vi "scanning_template_5_24.vi"() -> ()   [LabVIEW 2022 SP3]
uses:
  <vilib>/Utility/file.llb/Write Delimited Spreadsheet (string).vi
panel:
  in  "Backwards x":bool
  in  "ms to wait after move":u32=200
  in  "ANC300 address":refnum<visa-resource-name>="COM8"
  in  "Snake":bool
  in  "File to save to":path=path "C:/Users/Public/OneDrive/Desktop/test.txt"
  in  "Select Scan Type":u16(ring) items=["line scan", "rectangular scan"]
  in  "scan points":i32
  in  "y end":i32
  in  "x end":i32
  in  "y start":i32
  in  "x start":i32
  in  "y scan points":i32
  in  "x scan points":i32
  in  "y scan size":i32
  in  "x scan size":i32
  in  "y center":i32
  in  "x center":i32
  # "Scaning Setup"
  # "Rectangular Scan Parameters"
  # "Line Scan Parameters"
  # "Measurement Setup"
  # "insert measurement controls"
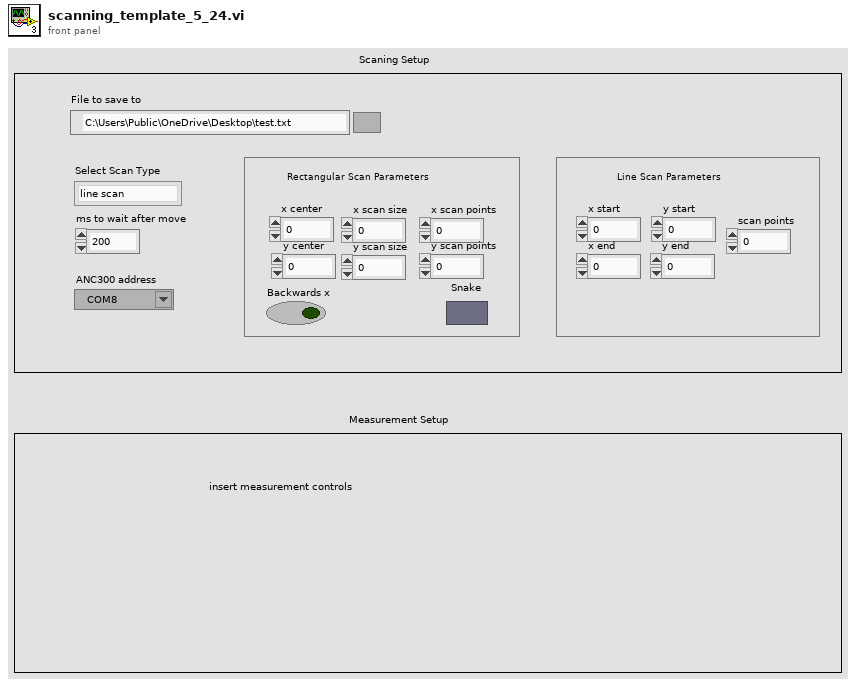
[diagram p1: front panel]
types:
  T1 = cluster{"error ":bool, "error number":i32, "error code":string}
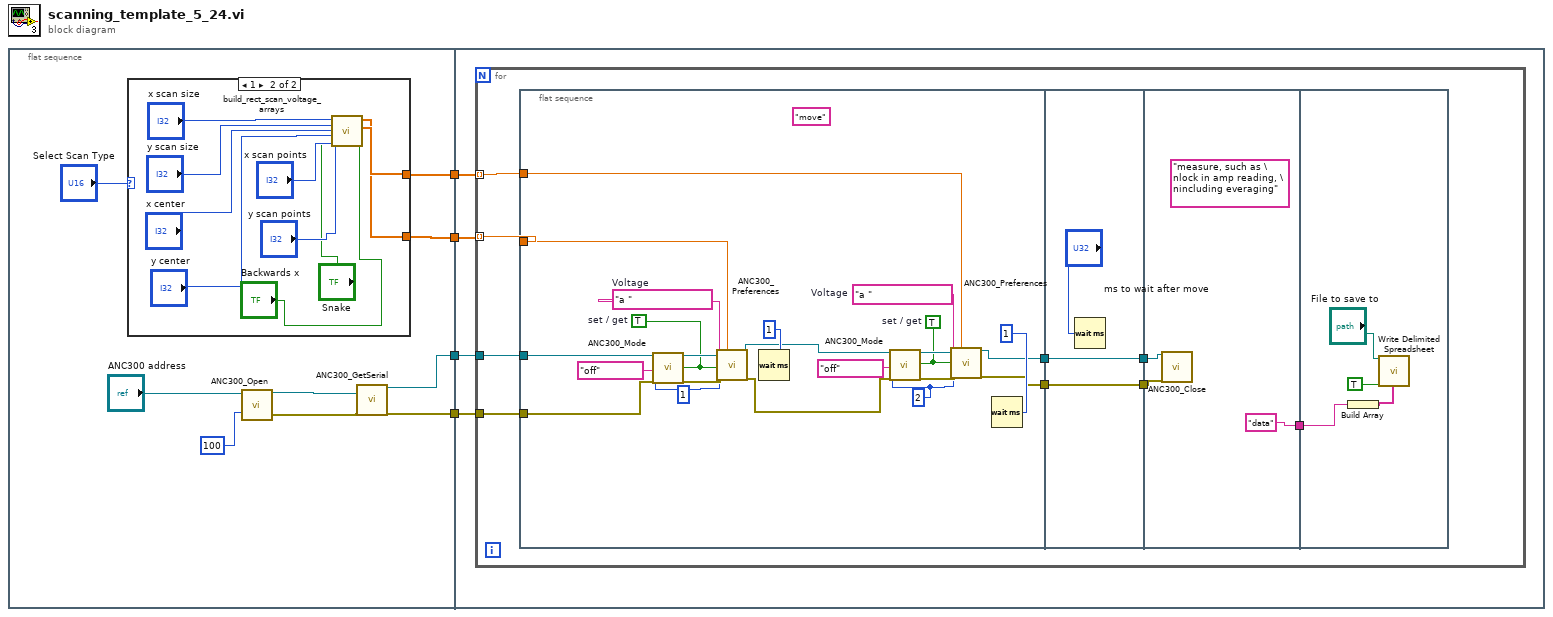
[diagram p0: block diagram]
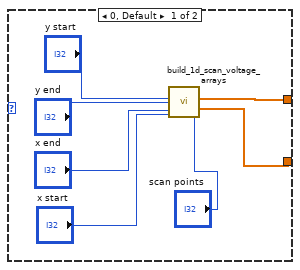
[diagram p2: hidden frame]
diagram:
  n1 = flat-sequence {
    tunnel: [w12] -> w4
    tunnel: [w13] -> w3
    tunnel: [w7] -> w2
    tunnel: [w6] -> w1
    tunnel: w4 -> [w34]
    tunnel: w3 -> [w33]
    tunnel: w2 -> [w32]
    tunnel: w1 -> [w31]
    frame #0 {
      n2 = case shown="1" "Select Scan Type" {
        tunnel: [w14 w30] -> w13
        tunnel: [w15 w29] -> w12
        frame 0, Default {
          n3 = call "build_1d_scan_voltage_arrays.vi"("y end"="y end", "y start"="y start", "scan points"="scan points", "x start"="x start", "x end"="x end") -> ("y voltage array"=w14:dbl[], "x voltage array"=w15:dbl[])  [unwired: 5 in]
        }
        frame 1 {
          n4 = call "build_rect_scan_voltage_arrays.vi"("Backwards x"="Backwards x", "y scan points"="y scan points", "y scan size"="y scan size", "x center"="x center", "Snake"="Snake", "y center"="y center", "x scan points"="x scan points", "x scan size"="x scan size") -> ("y voltage array"=w30:dbl[], "x voltage array"=w29:dbl[])  [unwired: 2 in]
        }
      }
      n5 = call "ANC300_Open.vi"("ANC300 Communication Port In"="ANC300 address", "milliseconds to wait"=u32 100 ("millisecond timer value")) -> ("ANC300 Communication Port Out"=w8:refnum<visa-resource-name>, "error out"=w5:T1)  [unwired: 13 in, 3 out]
      n6 = call "ANC300_GetSerial.vi"("ANC300 Communication Port In"=w8, "error in"=w5) -> ("ANC300 Communication Port Out"=w7:refnum<visa-resource-name>, "error out"=w6:T1)  [unwired: 10 in, 6 out]
    }
    frame #1 {
      n7 = for {
        tunnel: w34 -> [w43] mode=indexing
        tunnel: w33 -> [w42] mode=indexing
        tunnel: w32 -> [w41]
        tunnel: w31 -> [w40]
        n8 = flat-sequence {
          tunnel: w43 -> [w50]
          tunnel: w42 -> [w49]
          tunnel: w41 -> [w52]
          tunnel: w40 -> [w47]
          tunnel: [w45] -> w38
          tunnel: [w44] -> w37
          tunnel: w38 -> [w67]
          tunnel: w37 -> [w66]
          tunnel: [w67] -> w36
          tunnel: [w66] -> w35
          tunnel: ["data"] -> w39
          tunnel: w36 -> [w70]
          tunnel: w35 -> [w69]
          tunnel: w39 -> [w72]
          frame #0 {
            w53 = 2
            w54 = 1
            w55 = TRUE  # set / get
            w57 = "a "  # Voltage
            w60 = TRUE  # set / get
            w63 = "a "  # Voltage
            (unwired) "move"
            n9 = call "ANC300_Mode.vi"("ANC300 Communication Port In"=w52, "Axis"=w54, "axis mode in"="off", "error in"=w47, "set / get"=w60) -> ("ANC300 Communication Port Out"=w65:refnum<visa-resource-name>, "error out"=w64:T1)  [unwired: 8 in, 5 out]
            n10 = call "ANC300_Preferences.vi"("ANC300 Communication Port In"=w65, "Axis"=w54, "value in"=w50, "parameter"=w63, "error in"=w64, "set / get"=w60) -> ("ANC300 Communication Port Out"=w48:refnum<visa-resource-name>, "error out"=w46:T1)  [unwired: 6 in, 6 out]
            n11 = Wait (ms)(milliseconds to wait=u32 1 ("1: ms to wait")) -> ()  [unwired: 1 out]
            n12 = call "ANC300_Mode.vi"("ANC300 Communication Port In"=w48, "Axis"=w53, "axis mode in"="off", "error in"=w46, "set / get"=w55) -> ("ANC300 Communication Port Out"=w59:refnum<visa-resource-name>, "error out"=w58:T1)  [unwired: 8 in, 5 out]
            n13 = call "ANC300_Preferences.vi"("ANC300 Communication Port In"=w59, "Axis"=w53, "value in"=w49, "parameter"=w57, "error in"=w58, "set / get"=w55) -> ("ANC300 Communication Port Out"=w45:refnum<visa-resource-name>, "error out"=w44:T1)  [unwired: 6 in, 6 out]
            n14 = Wait (ms)(milliseconds to wait=u32 1 ("2: ms to wait")) -> ()  [unwired: 1 out]
          }
          frame #1 {
            n15 = Wait (ms)(milliseconds to wait="ms to wait after move") -> ()  [unwired: 1 out]
          }
          frame #2 {
            (unwired) "measure, such as \nlock in amp reading, \nincluding everaging"
            n16 = call "ANC300_Close.vi"("ANC300 Communication Port In"=w70, "error in"=w69) -> ()  [unwired: 17 in, 1 out]
          }
          frame #3 {
            n17 = Build Array(w72) -> (w75:string[])
            n18 = call-poly <vilib>:"Write Delimited Spreadsheet.vi"("file path (dialog if empty)"="File to save to", "1D data"=w75, "append to file? (new file:F)"=TRUE) -> ()  [unwired: 11 in, 2 out]
          }
        }
      }
    }
  }
